vi "instantiate class.vi"(8 "error in (no error)":errorcluster, 10 "Beverage to be wrapped.lvclass":refnum<class "Beverage.lvclass">, 11 "CondimentDecorator in":refnum<class "CondimentDecorator.lvclass">) -> (0 "error out":errorcluster, 3 "CondimentDecorator out":refnum<class "CondimentDecorator.lvclass">)   [LabVIEW 2021]
uses:
  CondimentDecorator.lvclass
  Beverage/Beverage.lvclass
  CondimentDecorator.lvclass/CondimentDecorator.ctl
panel:
  # "Connector Pane"
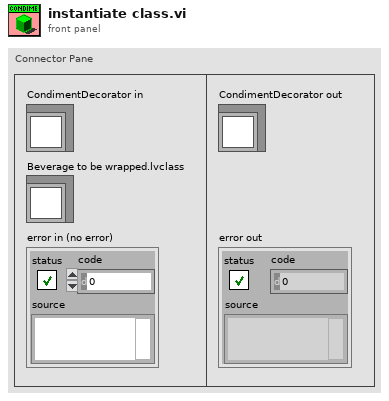
[diagram p1: front panel]
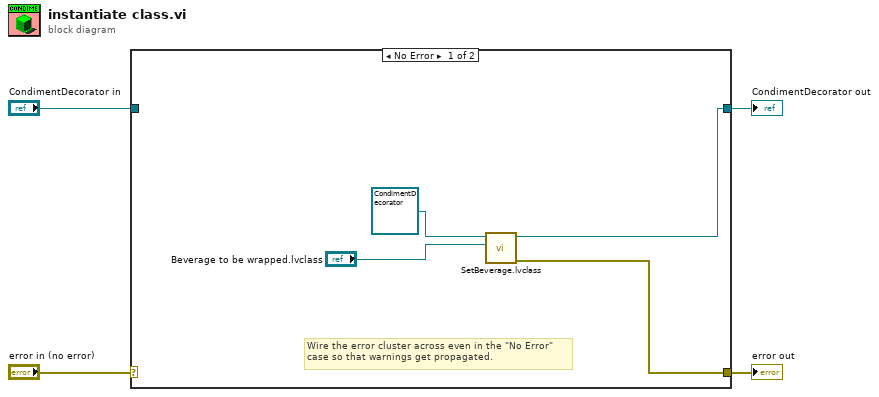
[diagram p0: block diagram]
diagram:
  n1 = case shown="No Error" "error in (no error)" {
    selector: "error in (no error)" -> [_ w10]
    tunnel: [w6 w10] -> w3
    tunnel: [w5 w9] -> w1
    tunnel: "CondimentDecorator in" -> [_ w9]
    frame No Error {
      # "Wire the error cluster across even in the \"No Error\"\ncase so that warnings get propagated."
      n2 = call-dynamic "SetBeverage.lvclass.vi"("Beverage.lvclass"="Beverage to be wrapped.lvclass", "object in"=refnum<class "CondimentDecorator.lvclass"> refnum ("CondimentDecorator.lvclass")) -> ("error out"=w6:errorcluster, "object out"=w5:refnum<class "CondimentDecorator.lvclass">)  [unwired: 8 in]
    }
    frame Error {
    }
  }
  "error out" <- w3
  "CondimentDecorator out" <- w1
